vi "String SW.vi"(11 "Data In":string) -> (3 "Data Out":string)   [LabVIEW 2016]
uses:
  Core/Assert API Components/Failure Actions.ctl
  Core/Assert API Components/Assert API Components.lvlib
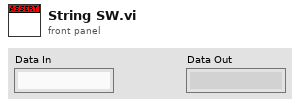
[diagram p1: front panel]
types:
  T1 = typedef "Assert API Components.lvlib/Failure Actions.ctl" = enum16{"None", "Log To File", "Pause Execution", "Abort Execution"}
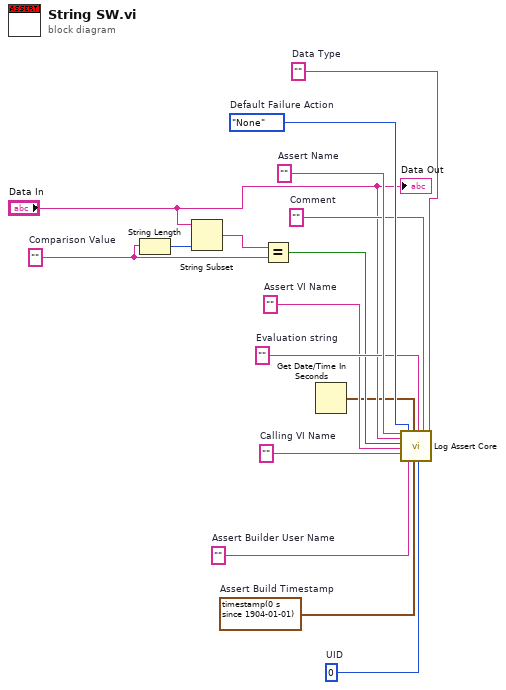
[diagram p0: block diagram]
diagram:
  w1 = 0  # UID
  w3 = ""  # Assert VI Name
  w4 = ""  # Calling VI Name
  w5 = ""  # Assert Builder User Name
  w6 = timestamp(0 s since 1904-01-01)  # Assert Build Timestamp
  w7 = ""  # Data Type
  w14 = ""  # Comment
  w13 = ""  # Evaluation string
  w15 = Failure_Actions."None"  # Default Failure Action
  w16 = ""  # Assert Name
  w9 = ""  # Comparison Value
  n1 = String Length(string=w9) -> (length=w11:i32)
  n2 = String Subset(string="Data In", length (rest)=w11) -> (substring=w10:string)  [unwired: 1 in]
  n3 = Equal?(x=w10, y=w9) -> (x = y?=w8:bool)
  n4 = Get Date/Time In Seconds() -> (seconds since 1Jan1904=w2:timestamp)
  n5 = call "Log Assert Core.vi"("Assert Name"=w16, "Data Value"="Data In", "Status"=w8, "Assert VI Name"=w3, "Calling VI Name"=w4, "Failure Action"=w15, "Assert Builder User Name"=w5, "Last Update"=w2, "Assert Build Timestamp"=w6, "Evaluation String"=w13, "Assert VI UID"=w1, "Comment"=w14, "Data Type"=w7) -> ()  [unwired: 7 in]
  "Data Out" <- "Data In"
